vi "360 Angle Calc.vi"(11 "Center":cluster{"X":dbl, "Y":dbl}) -> (3 "angle":dbl)   [LabVIEW 2025]
panel:
  in  "deg/pix":dbl=0.125
  out "X":dbl
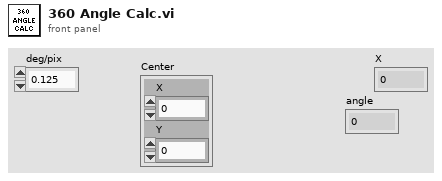
[diagram p1: front panel]
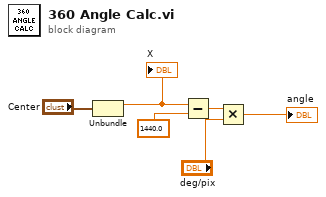
[diagram p0: block diagram]
diagram:
  n1 = Unbundle("Center") -> ("X"=w5:dbl)  [unwired: 1 out]
  "X" <- w5
  n2 = Subtract(x=w5, y=1440.0) -> (x-y=w3:dbl)
  n3 = Multiply(x=w3, y="deg/pix") -> (x*y=→"angle":dbl)
